vi "_CSTK_Button_Icon_Config_getInstalledFonts.vi"(8 "错误输入（无错误）":errorcluster) -> (0 "错误输出":errorcluster, 3 "已安装字体列表":string[](array[string]))   [LabVIEW 2015, in "CSTK_Button_Icon.xctl"]
uses:
  System.Drawing
  CSTK_Button_Icon.xctl
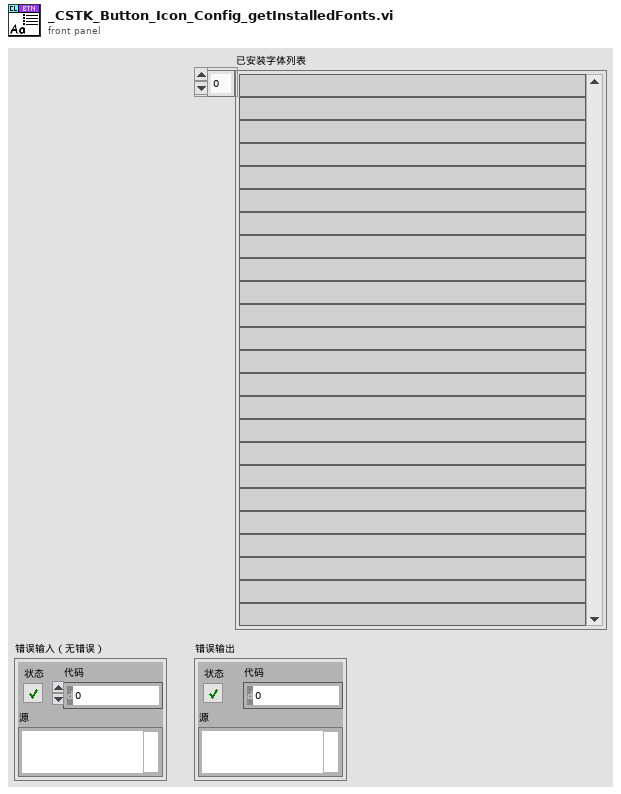
[diagram p1: front panel]
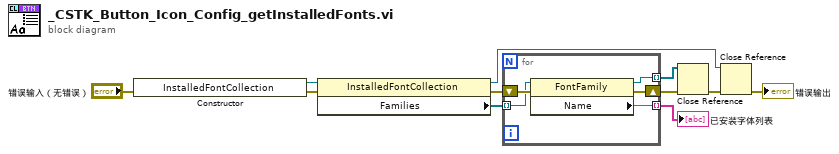
[diagram p0: block diagram]
diagram:
  n1 = constructor class="InstalledFontCollection"(error in="错误输入（无错误）") -> (reference out=w10:refnum<k24>, error out=w11:errorcluster)  [unwired: 2 in, 1 out]
  n2 = property class="InstalledFontCollection"(reference=w10, error in=w11) -> (reference out=w3:refnum<k24>, error out=w7:errorcluster, "Families"=w9:refnum<k24>[])
  n3 = for {
    tunnel: w9 -> [w12] mode=indexing
    tunnel: [w16] -> w8 mode=indexing
    shift-right: [w14] -> w5
    shift-left: w7 -> [w15]
    tunnel: [w13] -> w6 mode=indexing
    n4 = property class="FontFamily"(reference=w12, error in=w15) -> (reference out=w13:refnum<k24>, error out=w14:errorcluster, "Name"=w16:string)
  }
  "已安装字体列表" <- w8
  n5 = Close Reference(reference=w6, error in (no error)=w5) -> (error out=w4:errorcluster)
  n6 = Close Reference(reference=w3, error in (no error)=w4) -> (error out=→"错误输出":errorcluster)
